vi "reading string.vi"() -> ()   [LabVIEW 2020]
uses:
  <vilib>/Instr/_visa.llb/VISA Configure Serial Port (Instr).vi
panel:
  in  "data bits (8)":u16=8 min=5 max=8 step=1
  in  "baud rate (9600)":u32=9600
  in  "VISA resource name":refnum<visa-resource-name>
  out "error out 2":errorcluster
  out "read buffer":string
  out "error out":errorcluster
  out "return value":string
  in  "Enum":enum16{"Device A", "Device B", "UBD5"}(ring)
  out "Action":string
  out "millisecond timer value":u32
  in  "stop":bool
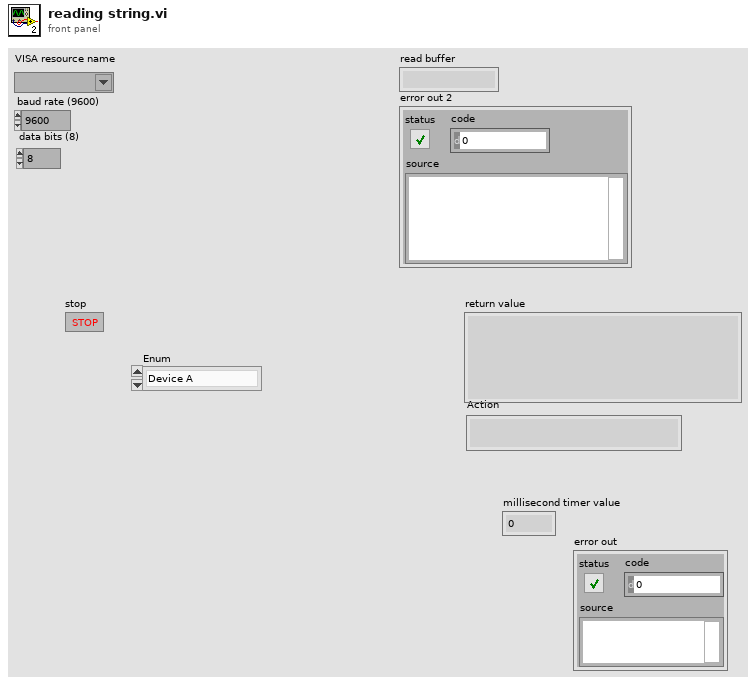
[diagram p1: front panel]
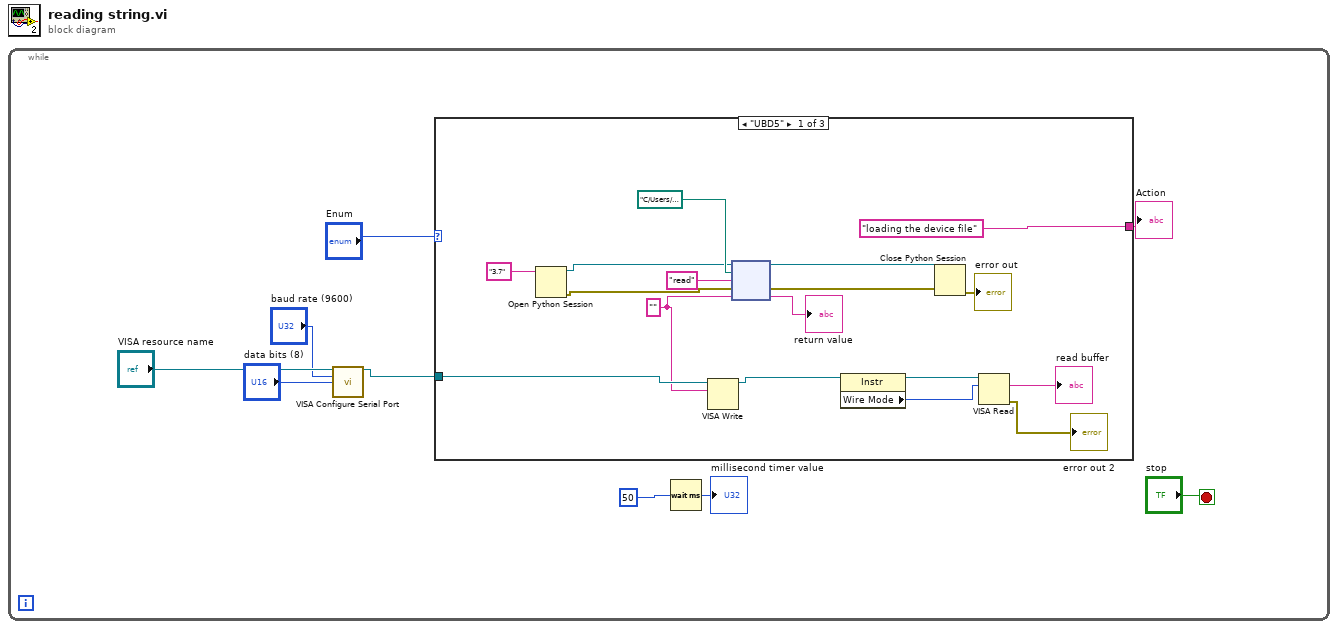
[diagram p0: block diagram]
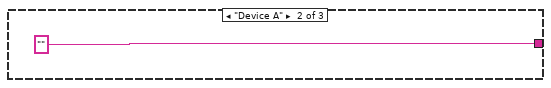
[diagram p2: hidden frame]
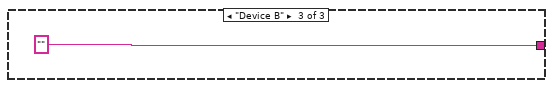
[diagram p3: hidden frame]
diagram:
  n1 = while {
    stop <- "stop" stop-if-true
    n2 = call-poly "VISA Configure Serial Port"("VISA resource name"="VISA resource name", "baud rate (9600)"="baud rate (9600)", "data bits (8)"="data bits (8)") -> ("VISA resource name out"=w4:refnum<visa-resource-name>)  [unwired: 11 in, 1 out]
    n3 = case shown="\"UBD5\"" "Enum" {
      tunnel: ["loading the device file" "" ""] -> w9
      tunnel: w4 -> [w12 _ _]
      frame "UBD5" {
        w11 = ""
        n4 = Open Python Session(python version="3.7" ("Python version")) -> (session out=w18:refnum<k35>, error out=w19:errorcluster)  [unwired: 2 in]
        n5 = VISA Write(VISA resource name=w12, write buffer=w11) -> (VISA resource name out=w16:refnum<visa-resource-name>)  [unwired: 1 in, 2 out]
        n6 = node(w18, path "C:/Users/battines/Documents/PycharmProjects/arrays.py" ("module path"), "read" ("function name"), w19, w11) -> (w25:refnum<k35>, w26:errorcluster, →"return value":string)  [unwired: 2 out]
        n7 = property class="Instr"(reference=w16) -> (reference out=w15:refnum<visa-resource-name>, "Wire Mode"=w14:i16)  [unwired: 1 in, 1 out]
        n8 = Close Python Session(session in=w25, error in=w26) -> (11:→"error out":errorcluster)
        n9 = VISA Read(VISA resource name=w15, byte count=w14) -> (read buffer=→"read buffer":string, error out=→"error out 2":errorcluster)  [unwired: 1 in, 2 out]
      }
      frame "Device A" {
      }
      frame "Device B" {
      }
    }
    "Action" <- w9
    n10 = Wait (ms)(milliseconds to wait=u32 50) -> (millisecond timer value=→"millisecond timer value":u32)
  }
